vi "SignalAttrbGet.vi"(0 "MessageFrame":refnum<k21>="ESP_1\nLRA110") -> (14 "SignalsNameArry":string[](array[string]), 15 "ScaleFac":dbl[](array[numeric]), 16 "StartBitArry":u32[](array[numeric]), 17 "Length":u32[](array[numeric]), 18 "DataType":u32[](array[numeric]), 19 "DefaultValue":dbl[](array[numeric]))   [LabVIEW 2020]
uses:
  <resource>/objmgr/xnet.rc
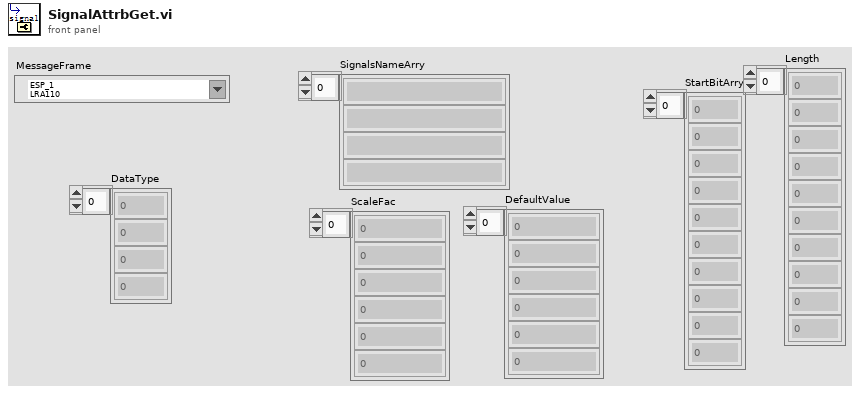
[diagram p1: front panel]
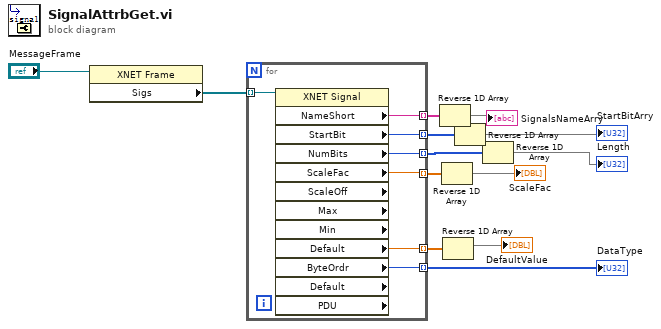
[diagram p0: block diagram]
diagram:
  n1 = property class="XNET Frame"(reference="MessageFrame") -> ("Sigs"=w12:refnum<k21>[])  [unwired: 1 in, 2 out]
  n2 = for {
    tunnel: w12 -> [w20] mode=indexing
    tunnel: [w19] -> w11 mode=indexing
    tunnel: [w18] -> w10 mode=indexing
    tunnel: [w17] -> w7 mode=indexing
    tunnel: [w16] -> w3 mode=indexing
    tunnel: [w15] -> w4 mode=indexing
    tunnel: [w14] -> w1 mode=indexing
    n3 = property class="XNET Signal" props=["NameShort", "StartBit", "NumBits", "ScaleFac", "ScaleOff", "Max", "Min", "Default", "ByteOrdr", "Default", "PDU"](reference=w20) -> ("NameShort"=w19:string, "StartBit"=w16:u32, "NumBits"=w14:u32, "ScaleFac"=w18:dbl, "Default"=w17:dbl, "ByteOrdr"=w15:u32)  [unwired: 1 in, 7 out]
  }
  "DataType" <- w4
  n4 = Reverse 1D Array(array=w11) -> (reversed array=→"SignalsNameArry":string[])
  n5 = Reverse 1D Array(array=w10) -> (reversed array=→"ScaleFac":dbl[])
  n6 = Reverse 1D Array(array=w7) -> (reversed array=→"DefaultValue":dbl[])
  n7 = Reverse 1D Array(array=w3) -> (reversed array=→"StartBitArry":u32[])
  n8 = Reverse 1D Array(array=w1) -> (reversed array=→"Length":u32[])
